vi "Read Log Session.vi"(8 "error in":errorcluster, 11 "Configurable Device in":refnum<class "Configurable Device.lvclass">) -> (0 "error out":errorcluster, 2 "Session Handle":T1, 3 "Configurable Device out":refnum<class "Configurable Device.lvclass">)   [LabVIEW 2015, in "Configurable Device.lvclass"]
uses:
  Configurable Device.lvclass
  <vilib>/MSR Consulting, LLC/General Reuse/Session APIs/_Session Fwk/Typedefs/Session Handle.ctl
  <vilib>/MSR Consulting, LLC/General Reuse/Session APIs/_Session Fwk/Session - Root.lvclass
  Configurable Device.lvclass/Configurable Device.ctl
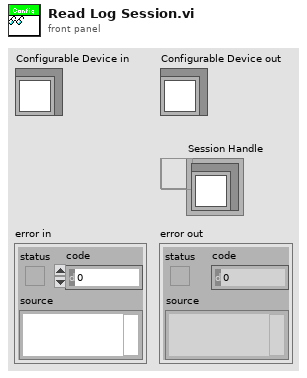
[diagram p1: front panel]
types:
  T1 = typedef "Session - Root.lvclass/Session Handle.ctl" = refnum<data-value>
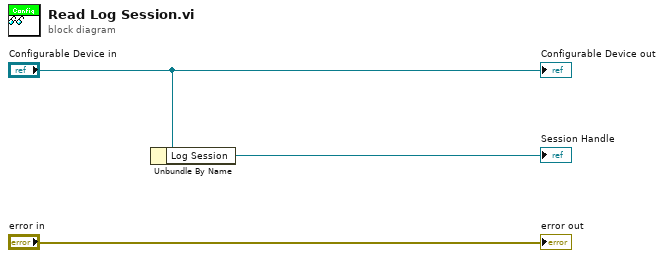
[diagram p0: block diagram]
diagram:
  n1 = Unbundle By Name("Configurable Device in") -> ("Log Session"=→"Session Handle":T1)
  "error out" <- "error in"
  "Configurable Device out" <- "Configurable Device in"
